vi "Configure Synchronization.vi"(0 "Register Buses":T1[](array[typedef]), 1 "scope":string(combo)="rx", 11 "error in":errorcluster) -> (4 "Register Buses (out)":T1[](array[typedef]), 15 "error out":errorcluster)   [LabVIEW 2017]
doc: "Configure and synchronize NI 579x devices.\n\n<B>Input Parameters</B>\n\n<B>Register Buses</B> specifies the Register Buses to which the Synchronization library is connected in the FPGA VIs.\n\n<B>scope</B> is the channel to configure synchronization for. The options are \"rx\" and \"tx\".\n\n<B>error in</B> describes error conditions that occur before this node runs. This input provides standard 'error in' functionality.\n\n<B>Output Parameters</B>\n\n<B>Register Buses (out)</B> passes the Register Buses to the next VI.\n\n<B>error out</B> contains error information. This output provides standard 'error out' functionality."
uses:
  <instrlib>/_niInstr/Register Bus/v0/Host/Public/Register Bus Session.ctl
  <instrlib>/_niInstr/Register Bus/v0/Host/Private/Session Data.ctl
  <vilib>/Utility/error.llb/Error Cluster From Error Code.vi
  <vilib>/rvi/errors/niLvFpgaAdjustHostInterfaceError.vi
  <vilib>/rvi/interface/nirviReadWriteControl/nirviReadWriteControl.xnode
  NiFpgaLv.dll
  <vilib>/rvi/interface/Simulation/niFpgaSimulationCallBeginRW.vi
  <instrlib>/ni579x/Synchronization/v2/Host/ni579x Synchronization v2 Host.lvlib
  <instrlib>/_niInstr/Register Bus/v0/Host/niInstr Register Bus v0 Host.lvlib
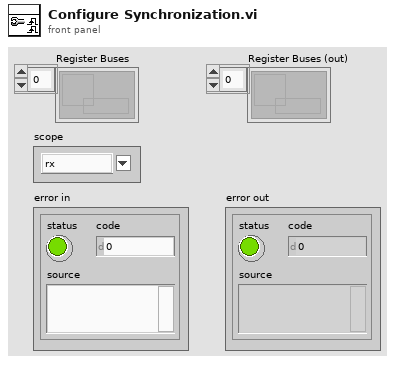
[diagram p1: front panel]
types:
  T1 = typedef "niInstr Register Bus v0 Host.lvlib/Register Bus Session.ctl" = refnum<queue>
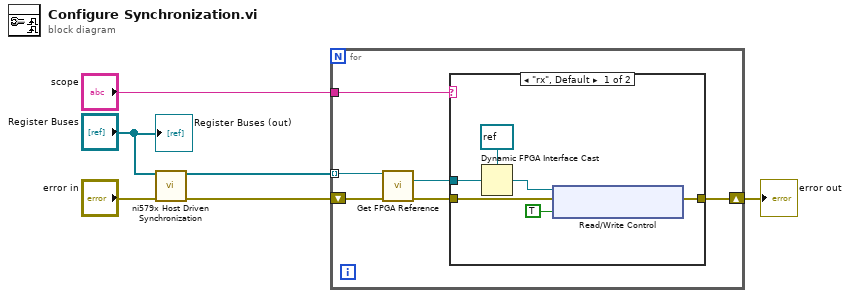
[diagram p0: block diagram]
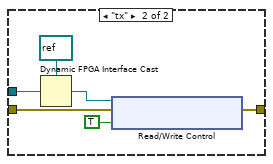
[diagram p2: hidden frame]
diagram:
  n1 = call <instrlib>:"ni579x Host Driven Synchronization.vi"("Register Buses"="Register Buses", "error in"="error in") -> ("Register Buses (out)"=w3:T1[], "error out"=w4:errorcluster)  [unwired: 12 in]
  n2 = for {
    tunnel: w3 -> [w12] mode=indexing
    shift-right: [w8] -> w5
    shift-left: w4 -> [w11]
    tunnel: "scope" -> [w7]
    n3 = call <instrlib>:"Get FPGA Reference.vi"("session in"=w12, "error in"=w11) -> ("fpga ref"=w9:refnum<k20>, "error out"=w10:errorcluster)  [unwired: 11 in, 1 out]
    n4 = case shown="\"rx\", Default" w7 {
      tunnel: w10 -> [w18 w24]
      tunnel: w9 -> [w16 w22]
      tunnel: [w13 w19] -> w8
      frame "rx", Default {
        n5 = Dynamic FPGA Interface Cast(Session In=refnum<k20> refnum ("Type"), Type=w16) -> (Session Out=w15:refnum<k20>)
        n6 = xnode "Read/Write Control"("FPGA VI Reference In"=w15, "error in"=w18, "rx.enable trigger sync"=TRUE ("rx.sw trigger.sync enable")) -> ("error out"=w13:errorcluster)  [unwired: 1 out]
      }
      frame "tx" {
        n7 = Dynamic FPGA Interface Cast(Session In=refnum<k20> refnum ("Type"), Type=w22) -> (Session Out=w21:refnum<k20>)
        n8 = xnode "Read/Write Control"("FPGA VI Reference In"=w21, "error in"=w24, "tx.enable trigger sync"=TRUE ("rx.sw trigger.sync enable")) -> ("error out"=w19:errorcluster)  [unwired: 1 out]
      }
    }
  }
  "error out" <- w5
  "Register Buses (out)" <- "Register Buses"
